vi "Configure FFT Measurement (Total Harmonic Distortion).vi"(7 "Fundamental Frequency (100000 Hz)":dbl=100000.0, 8 "error in (no error)":errorcluster, 9 "Track Mode (0: Auto)":i32(ring) items=["Auto", "Manual"], 10 "Measurement Source (0: Function 1)":i32(ring) items=["Function 1", "Function 2", "Function 3", "Function 4", "Math 1", "Math 2", "Math 3", "Math 4", "FFT"], 11 "VISA resource name":refnum<visa-resource-name>) -> (0 "error out":errorcluster, 3 "VISA resource name out":refnum<visa-resource-name>)   [LabVIEW 2017, in "Agilent 2000 3000 X-Series.lvlib"]
doc: "Configure FFT analysis total harmonic distortion (THD) measurement.\n\n<b>Note:</b>\n - This VI is only applicable for 3000T, 3000G, 4000, 6000 X-Series.\n - You need to call <b>Configure Math Function Source</b> set the signal source, and call <b>Configure Math Function Characteristics</b>set the function operation mode to FFT and turn on the display of the function."
uses:
  Agilent 2000 3000 X-Series.lvlib
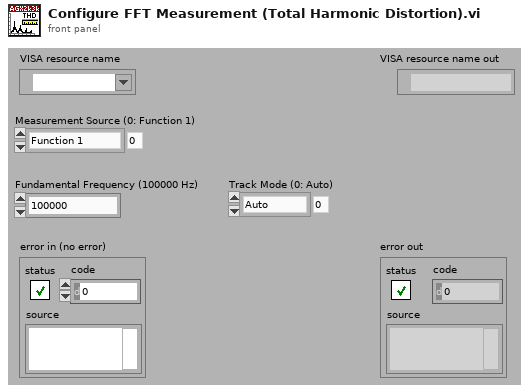
[diagram p1: front panel]
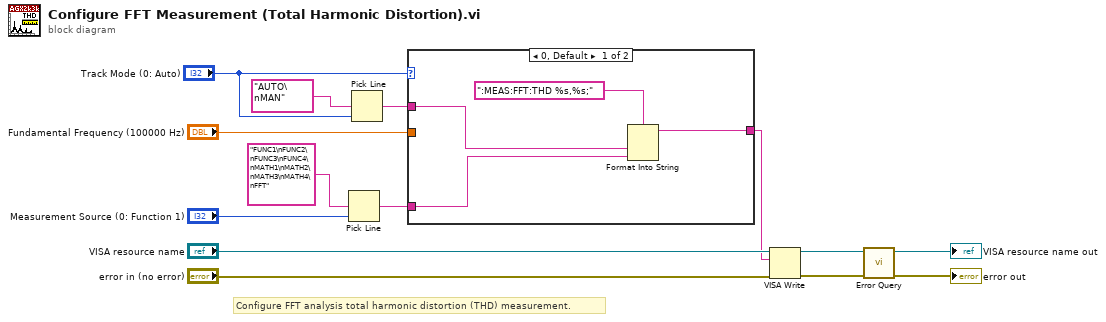
[diagram p0: block diagram]
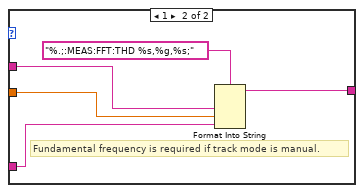
[diagram p2: hidden frame]
diagram:
  # "Configure FFT analysis total harmonic distortion (THD) measurement."
  n1 = Pick Line(multi-line string="FUNC1\nFUNC2\nFUNC3\nFUNC4\nMATH1\nMATH2\nMATH3\nMATH4\nFFT", line index="Measurement Source (0: Function 1)") -> (output string=w5:string)  [unwired: 1 in]
  n2 = Pick Line(multi-line string="AUTO\nMAN", line index="Track Mode (0: Auto)") -> (output string=w2:string)  [unwired: 1 in]
  n3 = case shown="0, Default" "Track Mode (0: Auto)" {
    tunnel: w5 -> [w16 w20]
    tunnel: "Fundamental Frequency (100000 Hz)" -> [_ w21]
    tunnel: w2 -> [w17 w22]
    tunnel: [w15 w19] -> w1
    frame 0, Default {
      n4 = Format Into String(format string=":MEAS:FFT:THD %s,%s;", w17, w16) -> (resulting string=w15:string)  [unwired: 2 in, 1 out]
    }
    frame 1 {
      # "Fundamental frequency is required if track mode is manual."
      n5 = Format Into String(format string="%.;:MEAS:FFT:THD %s,%g,%s;", w22, w21, w20) -> (resulting string=w19:string)  [unwired: 2 in, 1 out]
    }
  }
  n6 = VISA Write(VISA resource name="VISA resource name", write buffer=w1, error in (no error)="error in (no error)") -> (VISA resource name out=w9:refnum<visa-resource-name>, error out=w8:errorcluster)  [unwired: 1 out]
  n7 = call "Error Query.vi"("error in (no error)"=w8, "VISA resource name"=w9) -> ("error out"=→"error out":errorcluster, "VISA resource name out"=→"VISA resource name out":refnum<visa-resource-name>)  [unwired: 6 in, 2 out]
